vi "Manage_DOME.vi"() -> ()   [LabVIEW 2016]
uses:
  Manage_DOME/cgi_string.ctl
  <vilib>/Utility/miscctls.llb/LVComboBoxStrsAndValuesArrayTypeDef.ctl
  Manage_DOME/cgi_request.ctl
  <vilib>/httpClient/ClientHandle.ctl
  <vilib>/httpClient/LabVIEWHTTPClient.lvlib
panel:
  out "http_address":string
  out "finalStg":string
  in  "send":bool
  in  "Subst":string[](array[string]) caption="Substitution      ( string-->substitution )"
  out "Http string":string
  out "HEADER from Server":string
  in  "Remote host/IP address":string="84.253.163.35"
  in  "stop":bool
  in  "added_string":T1
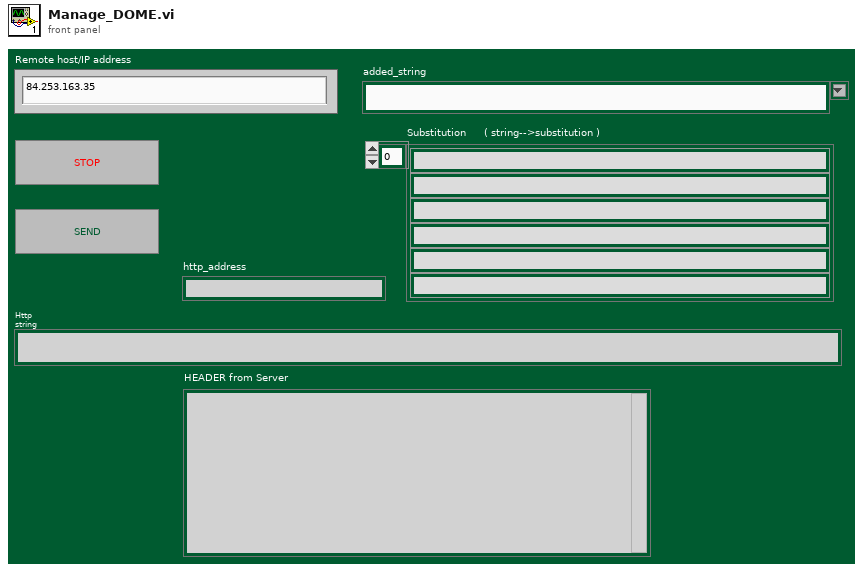
[diagram p1: front panel]
types:
  T1 = typedef "cgi_string.ctl" = string
  T2 = typedef "LVComboBoxStrsAndValuesArrayTypeDef.ctl" = cluster{"String":string, "Value":string}[]
  T3 = typedef "cgi_request.ctl" = cluster{"Client Handle":T4, "Exit":bool, "HttpStg":string}
  T4 = typedef "LabVIEWHTTPClient.lvlib/ClientHandle.ctl" = refnum<k1>
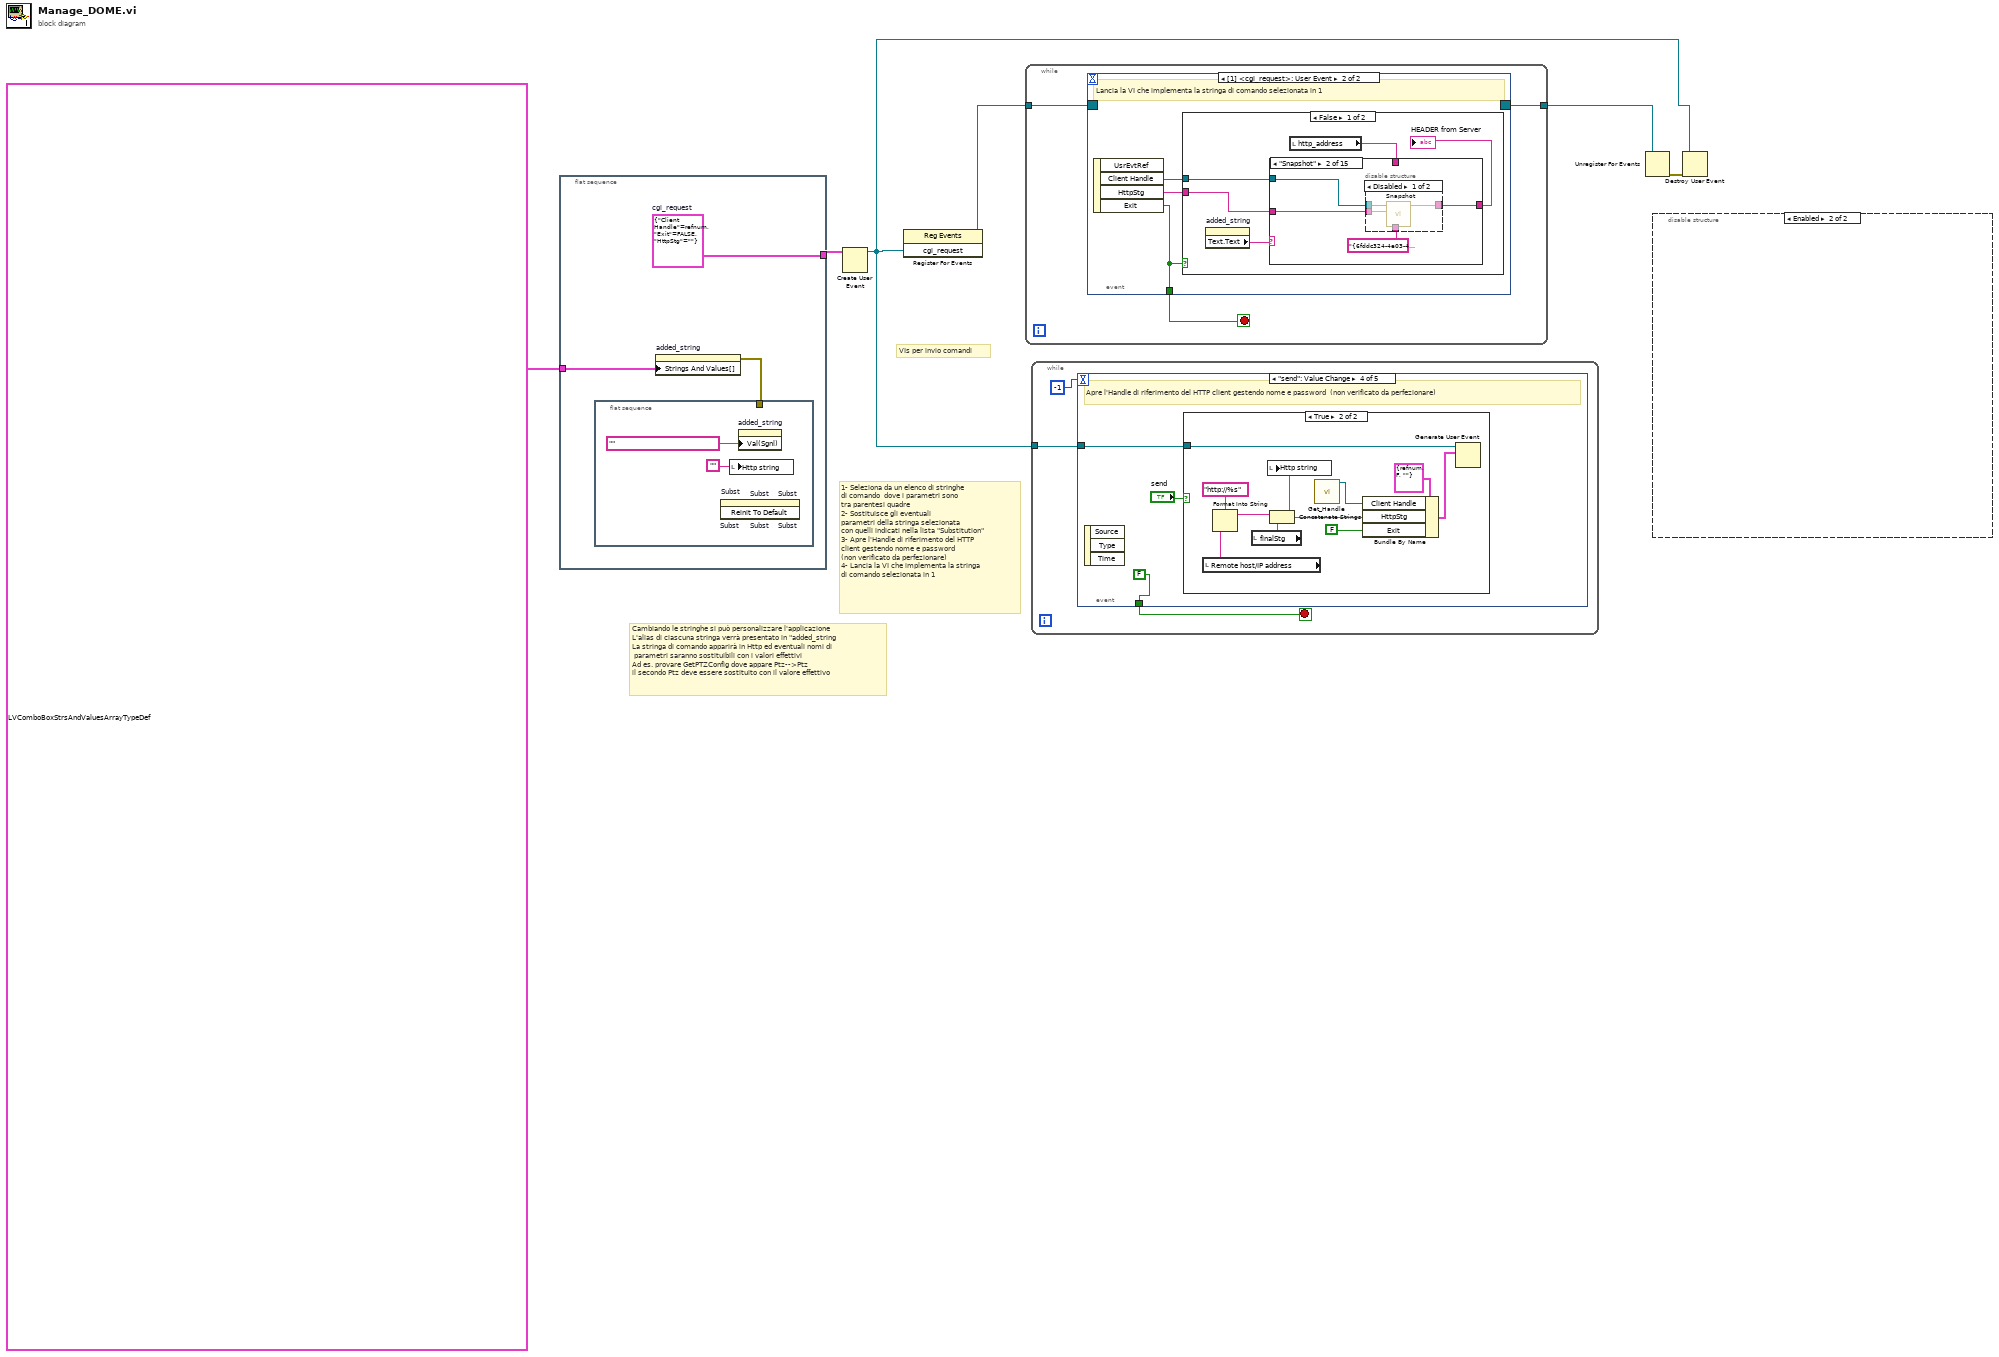
[diagram p0: block diagram]
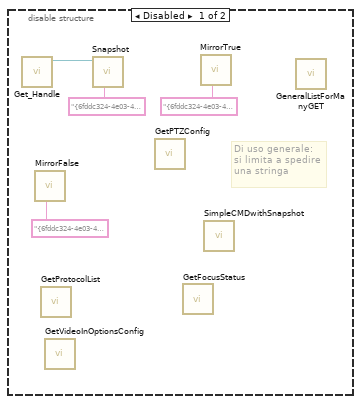
[diagram p2: hidden frame]
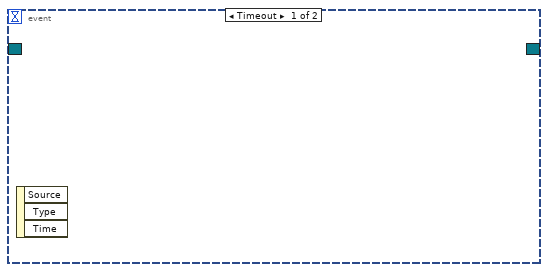
[diagram p3: hidden frame]
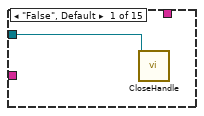
[diagram p4: hidden frame]
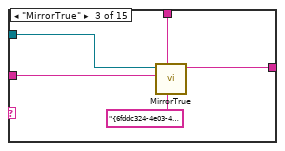
[diagram p6: hidden frame]
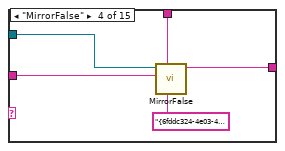
[diagram p7: hidden frame]
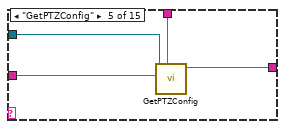
[diagram p8: hidden frame]
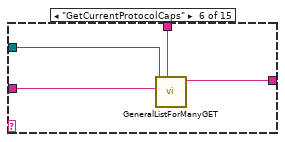
[diagram p9: hidden frame]
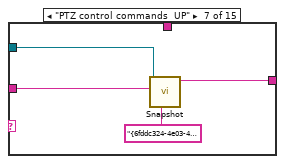
[diagram p10: hidden frame]
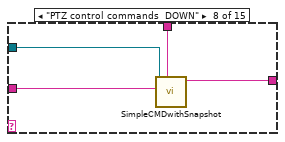
[diagram p11: hidden frame]
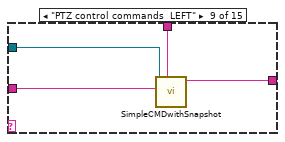
[diagram p12: hidden frame]
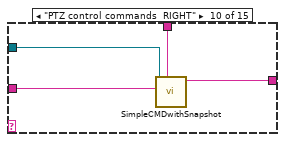
[diagram p13: hidden frame]
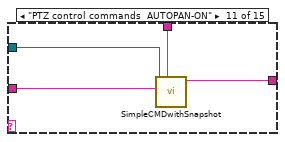
[diagram p14: hidden frame]
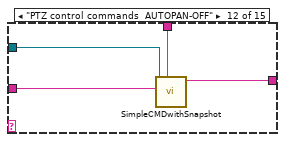
[diagram p15: hidden frame]
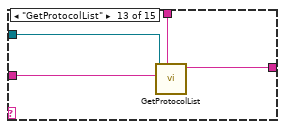
[diagram p16: hidden frame]
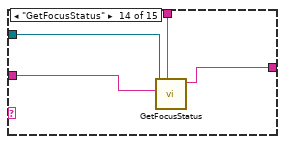
[diagram p17: hidden frame]
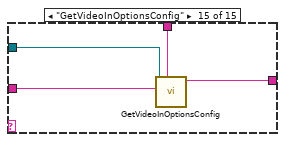
[diagram p18: hidden frame]
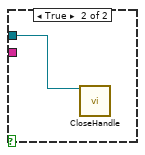
[diagram p19: hidden frame]
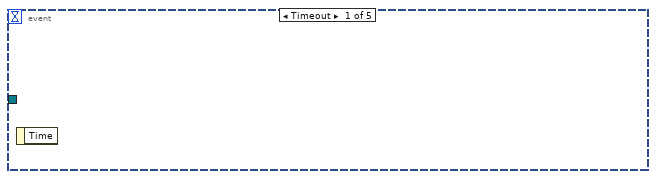
[diagram p20: hidden frame]
diagram:
  # "Cambiando le stringhe si può personalizzare l'applicazione\nL'alias di ciascuna stringa verrà presentato in \"added_string\nLa stringa di comando apparirà in Http ed eventuali nomi di \n parametri saranno sostituibili con i valori effettivi\nAd es. provare GetPTZConfig dove appare Ptz-->Ptz\nil secondo Ptz deve essere sostituito con il valore effettivo"
  # "VIs per invio comandi"
  # "1- Seleziona da un elenco di stringhe\ndi comando  dove i parametri sono\ntra parentesi quadre\n2- Sostituisce gli eventuali\nparametri della stringa selezionata \ncon quelli indicati nella lista \"Substitution\"\n3- Apre l'Handle di riferimento del HTTP\nclient gestendo nome e password \n(non verificato da perfezionare)\n4- Lancia la VI che implementa la stringa\ndi comando selezionata in 1"
  n1 = flat-sequence {
    tunnel: [w9] -> w6
    tunnel: T2 [{"String"="< select a string >", "Value"=""}, {"String"="GetVideoInOptionsConfig", "Value"="/cgi-bin/configManager.cgi?action=getConfig&name=VideoInOptions"}, {"String"="Snapshot", "Value"="/cgi-bin/snapshot.cgi?"}, {"String"="GetPTZConfig", "Value"="/cgi-bin/configManager.cgi?action=getConfig&name=Ptz"}, {"String"="MirrorTrue", "Value"="/cgi-bin/configManager.cgi?action=setConfig&VideoInOptions[0].Mirror=true"}, {"String"="MirrorFalse", "Value"="/cgi-bin/configManager.cgi?action=setConfig&VideoInOptions[0].Mirror=false"}, {"String"="GetProtocolList", "Value"="/cgi-bin/ptz.cgi?action=getProtocolList"}, {"String"="GetFocusStatus", "Value"="/cgi-bin/devVideoInput.cgi?action=getFocusStatus"}, {"String"="GetVideoStandardConfig", "Value"="/cgi-bin/configManager.cgi?action=getConfig&name=VideoStandard"}, {"String"="GetInterfaces  (NET)", "Value"="/cgi-bin/netApp.cgi?action=getInterfaces"}, {"String"="GetBasicConfig (NET Dns PhysAdd ....)", "Value"="/configManager.cgi?action=getConfig&name=Network"}, {"String"="GetPPPoEConfig", "Value"="/configManager.cgi?action=getConfig&name=PPPoE"}, {"String"="GetEmailConfig", "Value"="/configManager.cgi?action=getConfig&name=Email"}, {"String"="GetGeneralConfig", "Value"="/configManager.cgi?action=getConfig&name=General"}, {"String"="GetCurrentTime", "Value"="/cgi-bin/global.cgi?action=getCurrentTime"}, {"String"="GetGroupInfo", "Value"="/cgi-bin/userManager.cgi?action=getGroupInfo&name=admin"}, {"String"="GetUPnPConfig", "Value"="/cgi-bin/configManager.cgi?action=getConfig&name=UPnP"}, {"String"="GetNTPConfig", "Value"="/cgi-bin/configManager.cgi?action=getConfig&name=NTP"}, {"String"="GetRecordModeConfig", "Value"="/cgi-bin/configManager.cgi?action=getConfig&name=RecordMode"}, {"String"="GetNASConfig", "Value"="/cgi-bin/configManager.cgi?action=getConfig&name=NAS"}, {"String"="GetCurrentProtocolCaps", "Value"="/cgi-bin/ptz.cgi?action=getCurrentProtocolCaps&channel=<channelNo>"}, {"String"="PTZ control commands  UP", "Value"="/cgi-bin/ptz.cgi?action=start&channel=[ch]&code=Up&arg1=0& arg2=[argstr2]&arg3=0"}, {"String"="PTZ control commands  DOWN", "Value"="/cgi-bin/ptz.cgi?action=start&channel=[ch]&code=Down&arg1=0& arg2=[argstr2]&arg3=0"}, {"String"="PTZ control commands  LEFT", "Value"="/cgi-bin/ptz.cgi?action=start&channel=[ch]&code=left&arg1=0& arg2=[argstr2]&arg3=0"}, {"String"="PTZ control commands  RIGHT", "Value"="/cgi-bin/ptz.cgi?action=start&channel=[ch]&code=right&arg1=0& arg2=[argstr2]&arg3=0"}, {"String"="PTZ control commands  AUTOPAN-ON", "Value"="/cgi-bin/ptz.cgi?action=start&channel=[ch]&code=AutoPanOn&arg1=0& arg2=0&arg3=0"}, {"String"="PTZ control commands  AUTOPAN-OFF", "Value"="/cgi-bin/ptz.cgi?action=start&channel=[ch]&code=AutoPanOff&arg1=0& arg2=0&arg3=0"}] ("Strings And Values []") -> [w8]
    frame #0 {
      w9 = T3 {"Client Handle"=refnum, "Exit"=FALSE, "HttpStg"=""}  # cgi_request
      n2 = flat-sequence {
        tunnel: w7 -> [_]
        frame #0 {
          n3 = invoke on="Subst" class="Arr (strict)" method="Reinit To Default"() -> ()  [unwired: 3 in, 3 out]
          n4 = invoke on="Subst" class="Arr (strict)" method="Reinit To Default"() -> ()  [unwired: 3 in, 3 out]
          n5 = invoke on="Subst" class="Arr (strict)" method="Reinit To Default"() -> ()  [unwired: 3 in, 3 out]
          n6 = invoke on="Subst" class="Arr (strict)" method="Reinit To Default"() -> ()  [unwired: 3 in, 3 out]
          n7 = invoke on="Subst" class="Arr (strict)" method="Reinit To Default"() -> ()  [unwired: 3 in, 3 out]
          n8 = invoke on="Subst" class="Arr (strict)" method="Reinit To Default"() -> ()  [unwired: 3 in, 3 out]
          n9 = local write "Http string"("") -> ()
          n10 = property on="added_string" class="CmbBox (strict)"("Val(Sgnl)"=T1 "" ("added_string")) -> ()  [unwired: 2 in, 2 out]
        }
      }
      n11 = property on="added_string" class="CmbBox (strict)"("Strings And Values[]"=w8) -> (error out=w7:errorcluster)  [unwired: 2 in, 1 out]
    }
  }
  n12 = Create User Event(user event datatype=w6) -> (user event=w2:refnum<user-event>)  [unwired: 1 in, 1 out]
  n13 = register-events(w2) -> (reference out=w5:refnum<event-registration>)  [unwired: 2 in, 1 out]
  n14 = while {
    tunnel: w5 -> [w14]
    tunnel: [w13] -> w4
    stop <- w12 stop-if-true
    n15 = event shown="[1] <cgi_request>: User Event" {
      selector: w14 -> [_ _]
      dyn-events: [_ _] -> w13
      timeout: _ -> [_ _]
      tunnel: [_ w17] -> w12
      event Timeout {
        n16 = event-data() -> ()  [unwired: 1 in, 3 out]
      }
      event User Event {
        # "Lancia la VI che implementa la stringa di comando selezionata in 1"
        n17 = event-data() -> ("Client Handle"=w16:T4, "HttpStg"=w15:string, "Exit"=w17:bool)  [unwired: 1 in, 1 out]
        n18 = case shown="False" w17 {
          tunnel: w16 -> [w22 w86]
          tunnel: w15 -> [w20 _]
          frame False {
            n19 = property on="added_string" class="CmbBox (strict)"() -> ("Text.Text"=w18:string)  [unwired: 2 in, 2 out]
            n20 = local read "http_address"() -> (w19:string)
            n21 = case shown="\"Snapshot\"" w18 {
              tunnel: w20 -> [_ w26 w35 w40 w45 w49 w52 w57 w61 w65 w69 w73 w77 w81 w84]
              tunnel: w22 -> [w23 w27 w36 w41 w44 w48 w53 w56 w60 w64 w68 w72 w76 w80 w85]
              tunnel: [_ w24 w33 w38 w43 w47 w51 w55 w59 w63 w67 w71 w75 w79 w83] -> w21
              tunnel: w19 -> [_ _ w32 w37 w42 w46 _ w54 w58 w62 w66 w70 w74 w78 w82]
              frame "False", Default {
                n22 = call <vilib>:"CloseHandle.vi"("client handle"=w23) -> ()  [unwired: 14 in, 1 out]
              }
              frame "Snapshot" {
                n23 = disable-structure shown="Disabled" {
                  disable-tunnel: w27 -> [w31 _]
                  disable-tunnel: w26 -> [w30 _]
                  disable-tunnel: "{6fddc324-4e03-4bfe-b185-3d77768dc90e}" ("Dest Format") -> [w29 _]
                  disable-tunnel: [w28 _] -> w24
                  frame Disabled {
                    n24 = call "Snapshot.vi"("Dest Format"=w29, "Value"=w30, "Refnum in"=w31) -> ("headers"=w28:string)  [unwired: 8 in]
                  }
                  frame Enabled {
                  }
                }
              }
              frame "MirrorTrue" {
                n25 = call "MirrorTrue.vi"("Dest Format"="{6fddc324-4e03-4bfe-b185-3d77768dc90e}", "HTTP_address"=w32, "Value"=w35, "Refnum in"=w36) -> ("headers"=w33:string)  [unwired: 7 in]
              }
              frame "MirrorFalse" {
                n26 = call "MirrorFalse.vi"("Dest Format"="{6fddc324-4e03-4bfe-b185-3d77768dc90e}", "HTTP_address"=w37, "Value"=w40, "Refnum in"=w41) -> ("headers"=w38:string)  [unwired: 7 in]
              }
              frame "GetPTZConfig" {
                n27 = call "GetPTZConfig.vi"("HTTP_address"=w42, "Value"=w45, "Refnum in"=w44) -> ("headers"=w43:string)  [unwired: 7 in, 1 out]
              }
              frame "GetCurrentProtocolCaps" {
                n28 = call "GeneralListForManyGET.vi"("HTTP_address"=w46, "Value"=w49, "Refnum in"=w48) -> ("headers"=w47:string)  [unwired: 7 in, 1 out]
              }
              frame "PTZ control commands  UP" {
                n29 = call "Snapshot.vi"("Dest Format"="{6fddc324-4e03-4bfe-b185-3d77768dc90e}", "Value"=w52, "Refnum in"=w53) -> ("headers"=w51:string)  [unwired: 8 in]
              }
              frame "PTZ control commands  DOWN" {
                n30 = call "SimpleCMDwithSnapshot.vi"("HTTP_address"=w54, "Value"=w57, "Refnum in"=w56) -> ("headers"=w55:string)  [unwired: 8 in]
              }
              frame "PTZ control commands  LEFT" {
                n31 = call "SimpleCMDwithSnapshot.vi"("HTTP_address"=w58, "Value"=w61, "Refnum in"=w60) -> ("headers"=w59:string)  [unwired: 8 in]
              }
              frame "PTZ control commands  RIGHT" {
                n32 = call "SimpleCMDwithSnapshot.vi"("HTTP_address"=w62, "Value"=w65, "Refnum in"=w64) -> ("headers"=w63:string)  [unwired: 8 in]
              }
              frame "PTZ control commands  AUTOPAN-ON" {
                n33 = call "SimpleCMDwithSnapshot.vi"("HTTP_address"=w66, "Value"=w69, "Refnum in"=w68) -> ("headers"=w67:string)  [unwired: 8 in]
              }
              frame "PTZ control commands  AUTOPAN-OFF" {
                n34 = call "SimpleCMDwithSnapshot.vi"("HTTP_address"=w70, "Value"=w73, "Refnum in"=w72) -> ("headers"=w71:string)  [unwired: 8 in]
              }
              frame "GetProtocolList" {
                n35 = call "GetProtocolList.vi"("HTTP_address"=w74, "Value"=w77, "Refnum in"=w76) -> ("headers"=w75:string)  [unwired: 6 in, 2 out]
              }
              frame "GetFocusStatus" {
                n36 = call "GetFocusStatus.vi"("HTTP_address"=w78, "Value"=w81, "Refnum in"=w80) -> ("headers"=w79:string)  [unwired: 6 in, 2 out]
              }
              frame "GetVideoInOptionsConfig" {
                n37 = call "GetVideoInOptionsConfig.vi"("HTTP_address"=w82, "Value"=w84, "Refnum in"=w85) -> ("headers"=w83:string)  [unwired: 7 in, 1 out]
              }
            }
            "HEADER from Server" <- w21
          }
          frame True {
            n38 = call <vilib>:"CloseHandle.vi"("client handle"=w86) -> ()  [unwired: 14 in, 1 out]
          }
        }
      }
    }
  }
  n39 = while {
    tunnel: w2 -> [w88]
    stop <- w87 stop-if-true
    n40 = event shown="[3] \"send\": Value Change" {
      selector: _ -> [_ _ _ _ _]
      dyn-events: _ -> [_ _ _ _ _]
      timeout: -1 -> [_ _ _ _ _]
      tunnel: w88 -> [_ _ _ w135 w148]
      tunnel: [_ FALSE ("NewVal") _ FALSE w147] -> w87
      event Timeout {
        n41 = event-data() -> ()  [unwired: 1 in, 1 out]
      }
      event Value Change {
        # "Seleziona da un elenco di stringhe"
        n42 = event-data() -> ("NewVal"=w99:T1, "OldVal"=w100:T1)  [unwired: 1 in]
        n43 = local read "Subst"() -> (w101:string[])
        n44 = Not Equal?(x=w99, y=w100) -> (x != y?=w96:bool)
        n45 = for {
          tunnel: w101 -> [w110] mode=indexing
          shift-right: [w107] -> w92
          shift-left: "added_string" -> [w111]
          n46 = Match Pattern(string=w110, regular expression="-->") -> (before substring=w109:string, after substring=w108:string)  [unwired: 1 in, 2 out]
          n47 = Search and Replace String(input string=w111, search string=w109, replace string=w108) -> (result string=w107:string)  [unwired: 5 in, 3 out]
        }
        "finalStg" <- w92
        n48 = Not(x=w96) -> (.not. x?=w95:bool)
        n49 = control-ref of="added_string"() -> (w97:refnum<vi>)
        n50 = control-ref of="Subst"() -> (w98:refnum<vi>)
        n51 = Format Into String(format string="http://%s", "Remote host/IP address") -> (resulting string=w90:string)  [unwired: 2 in, 1 out]
        "http_address" <- w90
        n52 = call "UpdateParameterList.vi"("added_string"=w97, "Boolean"=w96, "Subst"=w98) -> ()  [unwired: 9 in]
        n53 = Concatenate Strings(w90, w92) -> (w91:string)
        n54 = Concatenate Strings(w90, "added_string") -> (w94:string)
        n55 = Select(t=w91, s=w95, f=w94) -> (s? t:f=→"Http string":string)
      }
      event "Subst": Value Change {
        # "Sostituisce gli eventuali parametri della stringa selezionata"
        n56 = event-data() -> ("NewVal"=w113:string[], "OldVal"=w114:string[])  [unwired: 1 in]
        n57 = for {
          tunnel: w114 -> [w123] mode=indexing
          tunnel: w113 -> [w125] mode=indexing
          tunnel: [w122] -> w112 mode=indexing
          n58 = Match Pattern(string=w123, regular expression="-->") -> (after substring=w121:string, offset past match=w119:i32)  [unwired: 1 in, 2 out]
          n59 = Add(x=w119, y=0) -> (x+y=w117:i32)
          n60 = Match Pattern(string=w125, regular expression="-->") -> (after substring=w124:string, offset past match=w118:i32)  [unwired: 1 in, 2 out]
          n61 = case shown="0, Default" w118 {
            tunnel: w124 -> [w132 _]
            tunnel: w123 -> [w131 w133]
            tunnel: [w130 w133] -> w122
            tunnel: w121 -> [w129 _]
            tunnel: w117 -> [w128 _]
            frame 0, Default {
              n62 = Search and Replace String(input string=w131, search string=w129, replace string=w132, offset=w128) -> (result string=w130:string)  [unwired: 4 in, 3 out]
            }
            frame -1 {
            }
          }
        }
        n63 = control-ref of="added_string"() -> (w115:refnum<vi>)
        n64 = local write "Subst"(w112) -> ()
        n65 = property class="CmbBox"(reference=w115) -> ("Value"=w116:string)  [unwired: 1 in, 2 out]
        n66 = property on="Property Node" class="CmbBox"(reference=w115, "Val(Sgnl)"=w116) -> ()  [unwired: 1 in, 2 out]
      }
      event "send": Value Change {
        # "Apre l'Handle di riferimento del HTTP client gestendo nome e password  (non verificato da perfezionare)"
        n67 = event-data() -> ()  [unwired: 1 in, 3 out]
        n68 = case shown="True" "send" {
          tunnel: w135 -> [_ w142]
          frame False {
          }
          frame True {
            n69 = local read "Remote host/IP address"() -> (w137:string)
            n70 = Format Into String(format string="http://%s", w137) -> (resulting string=w141:string)  [unwired: 2 in, 1 out]
            n71 = local read "finalStg"() -> (w138:string)
            n72 = Concatenate Strings(w141, w138) -> (w139:string)
            n73 = local write "Http string"(w139) -> ()
            n74 = call "Get_Handle.vi"() -> ("Refnum out"=w145:T4)  [unwired: 11 in]
            n75 = Bundle By Name(cluster=T3 {"Client Handle"=refnum, "Exit"=FALSE, "HttpStg"=""}, "Client Handle"=w145, "HttpStg"=w139, "Exit"=FALSE) -> (w144:T3)
            n76 = Generate User Event(user event=w142, event data cluster=w144) -> ()  [unwired: 2 in, 2 out]
          }
        }
      }
      event "stop": Value Change {
        n77 = event-data() -> ("NewVal"=w147:bool)  [unwired: 1 in]
        n78 = case shown="True" w147 {
          selector: w147 -> [_ w149]
          tunnel: w148 -> [_ w151]
          frame False {
          }
          frame True {
            n79 = call "Get_Handle.vi"() -> ("Refnum out"=w150:T4)  [unwired: 11 in]
            n80 = Bundle By Name(cluster=T3 {"Client Handle"=refnum, "Exit"=FALSE, "HttpStg"=""}, "Exit"=w149, "Client Handle"=w150) -> (w152:T3)
            n81 = Generate User Event(user event=w151, event data cluster=w152) -> ()  [unwired: 2 in, 2 out]
          }
        }
      }
    }
  }
  n82 = Unregister For Events(event registration refnum=w4) -> (error out=w3:errorcluster)  [unwired: 1 in]
  n83 = disable-structure shown="Enabled" {
    frame Disabled {
      # "Di uso generale:\nsi limita a spedire\nuna stringa"
      n84 = call "Get_Handle.vi"() -> ("Refnum out"=w154:T4)  [unwired: 11 in]
      n85 = call "MirrorFalse.vi"("Dest Format"="{6fddc324-4e03-4bfe-b185-3d77768dc90e}") -> ()  [unwired: 10 in, 1 out]
      n86 = call "GetProtocolList.vi"() -> ()  [unwired: 9 in, 3 out]
      n87 = call "GetVideoInOptionsConfig.vi"() -> ()  [unwired: 10 in, 2 out]
      n88 = call "Snapshot.vi"("Dest Format"="{6fddc324-4e03-4bfe-b185-3d77768dc90e}", "Refnum in"=w154) -> ()  [unwired: 9 in, 1 out]
      n89 = call "GetPTZConfig.vi"() -> ()  [unwired: 10 in, 2 out]
      n90 = call "GetFocusStatus.vi"() -> ()  [unwired: 9 in, 3 out]
      n91 = call "MirrorTrue.vi"("Dest Format"="{6fddc324-4e03-4bfe-b185-3d77768dc90e}") -> ()  [unwired: 10 in, 1 out]
      n92 = call "SimpleCMDwithSnapshot.vi"() -> ()  [unwired: 11 in, 1 out]
      n93 = call "GeneralListForManyGET.vi"() -> ()  [unwired: 10 in, 2 out]
    }
    frame Enabled {
    }
  }
  n94 = Destroy User Event(user event=w2, error in=w3) -> ()  [unwired: 1 out]
